vi "Finite_acq_gen_3.vi"(4 "Stimulator":T1={"frequency (Hz)"=1.0, "initial delay (ms)"=0.0, "# Stimuli"=0, "ON-OFF"=FALSE, "duty ratio"=0.0} {"frequency (Hz)" min=0.5 max=16.0 step=0.5 scale=0.0..10.0}, 5 "Shutter #2":T3={"Duration (ms)"=10.0, "Delay (ms)"=100.0, "# Cycles"=1, "period (ms)"=500.0, "ENABLE"=FALSE}, 6 "TRG detector":T2={"Delay (ms)"=100.0, "Duration (ms)"=1000.0, "ENABLE"=FALSE}, 7 "Shutter #1":T3={"Duration (ms)"=10.0, "Delay (ms)"=100.0, "# Cycles"=1, "period (ms)"=500.0, "ENABLE"=FALSE}, 8 "error in":errorcluster, 9 "samples per channel":i32=1000, 10 "ms/point":dbl=1.0, 11 "data":dbl[](array[numeric]) format="%0.2f") -> (3 "data 2":waveform(dbl)[](array[waveform]))   [LabVIEW 2011]
uses:
  <vilib>/DAQmx/write.llb/DAQmx Write (Analog 1D DBL 1Chan NSamp).vi
  <vilib>/DAQmx/read.llb/DAQmx Read (Analog 1D Wfm NChan NSamp).vi
  <vilib>/DAQmx/create/channels.llb/DAQmx Create Channel (AI-Voltage-Basic).vi
  <vilib>/DAQmx/configure/timing.llb/DAQmx Timing (Sample Clock).vi
  <vilib>/DAQmx/configure/trigger.llb/DAQmx Start Trigger (None).vi
  <vilib>/DAQmx/create/channels.llb/DAQmx Create Channel (CO-Pulse Generation-Frequency).vi
  <vilib>/DAQmx/configure/timing.llb/DAQmx Timing (Implicit).vi
  <vilib>/DAQmx/configure/trigger.llb/DAQmx Start Trigger (Digital Edge).vi
  <vilib>/DAQmx/create/channels.llb/DAQmx Create Channel (AO-Voltage-Basic).vi
  <vilib>/DAQmx/miscellaneous.llb/DAQmx Fill In Error Info.vi
  <vilib>/DAQmx/create/channels.llb/DAQmx Create Channel (CO-Pulse Generation-Time).vi
panel:
  # "STIMULATOR"
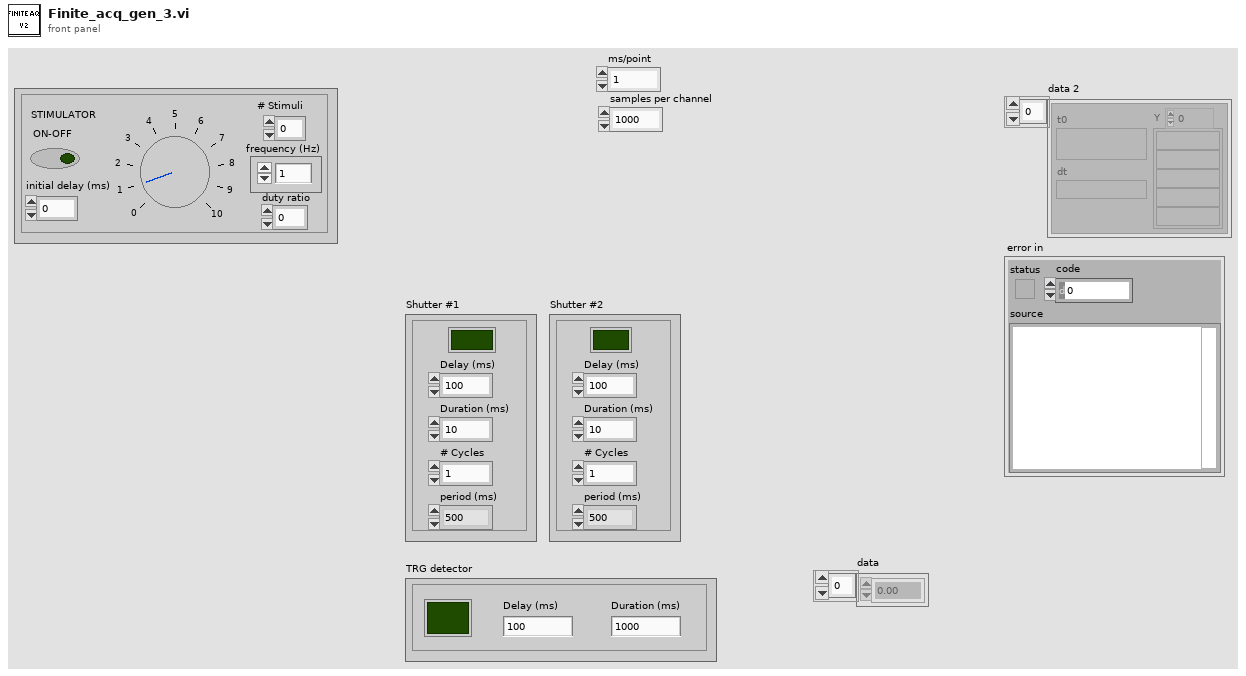
[diagram p1: front panel]
types:
  T1 = cluster{"frequency (Hz)":dbl, "initial delay (ms)":dbl, "# Stimuli":i8, "ON-OFF":bool, "duty ratio":dbl}
  T2 = cluster{"Delay (ms)":dbl, "Duration (ms)":dbl, "ENABLE":bool}
  T3 = cluster{"Duration (ms)":dbl, "Delay (ms)":dbl, "# Cycles":i8, "period (ms)":dbl, "ENABLE":bool}
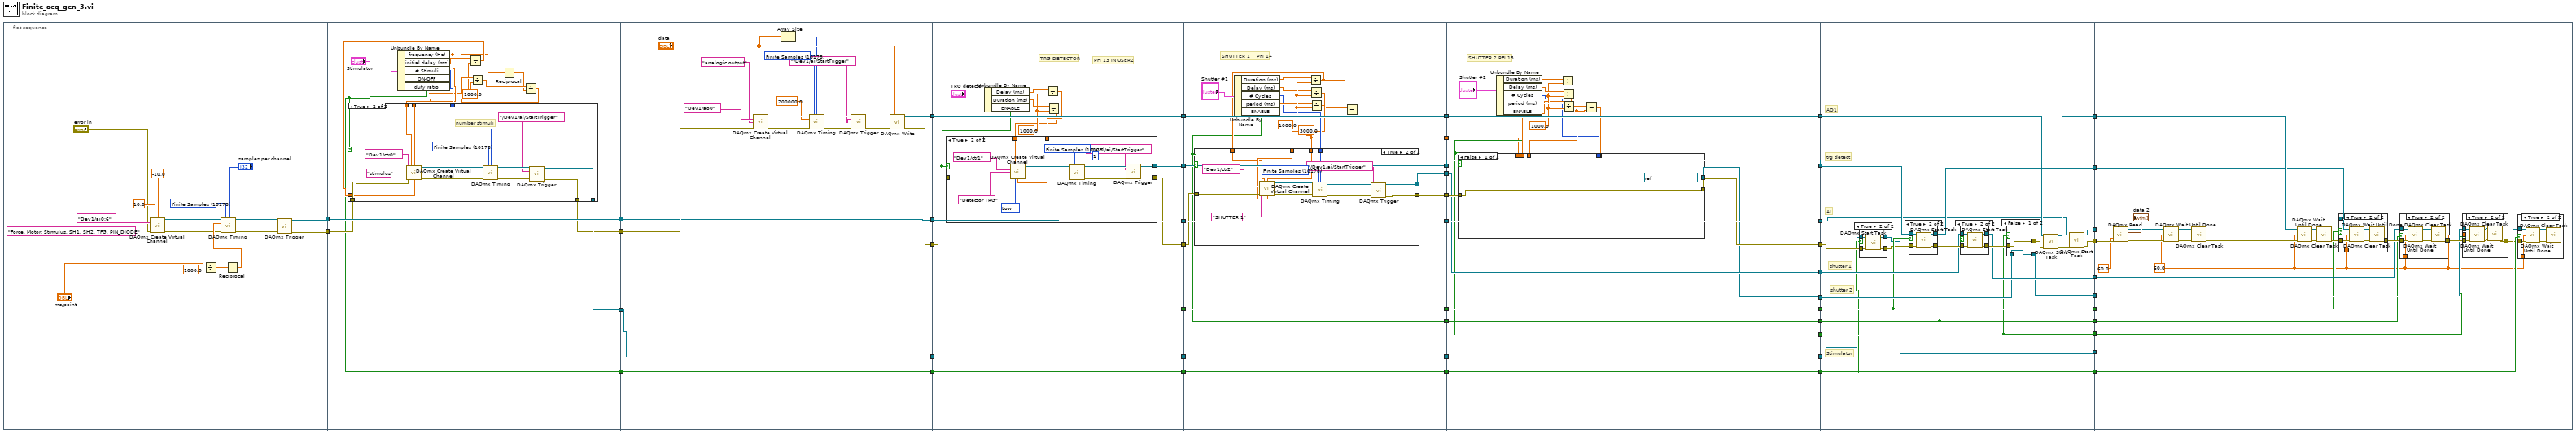
[diagram p0: block diagram]
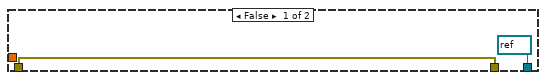
[diagram p2: hidden frame]
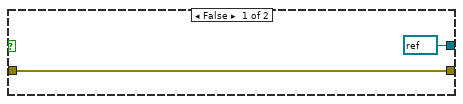
[diagram p3: hidden frame]
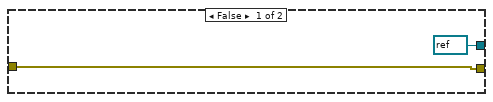
[diagram p4: hidden frame]
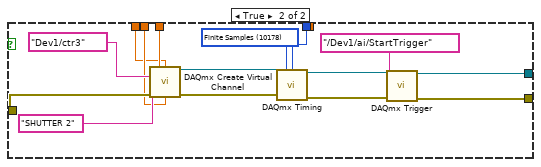
[diagram p5: hidden frame]
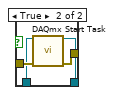
[diagram p7: hidden frame]
diagram:
  n1 = flat-sequence {
    tunnel: [w54] -> w16
    tunnel: [w52] -> w14
    tunnel: w16 -> [w81]
    tunnel: [w79] -> w15
    tunnel: w14 -> [w82]
    tunnel: [w82] -> w13
    tunnel: [w80] -> w8
    tunnel: [w75] -> w6
    tunnel: [w108] -> w48
    tunnel: [w113] -> w47
    tunnel: w15 -> [w109]
    tunnel: w13 -> [w108]
    tunnel: [w107] -> w46
    tunnel: [w101] -> w9
    tunnel: w8 -> [w101]
    tunnel: w6 -> [w100]
    tunnel: [w100] -> w5
    tunnel: w48 -> [w132]
    tunnel: [w132] -> w44
    tunnel: w47 -> [w128]
    tunnel: [w128] -> w43
    tunnel: w46 -> [w131]
    tunnel: [w130] -> w42
    tunnel: [w129] -> w41
    tunnel: [w121] -> w24
    tunnel: [w120] -> w10
    tunnel: w9 -> [w120]
    tunnel: w5 -> [w119]
    tunnel: [w119] -> w4
    tunnel: w44 -> [w169]
    tunnel: [w169] -> w40
    tunnel: w43 -> [w168]
    tunnel: [w168] -> w38
    tunnel: w42 -> [w166]
    tunnel: w41 -> [w167]
    tunnel: [w167] -> w35
    tunnel: [w165] -> w33
    tunnel: [w164] -> w31
    tunnel: [w154] -> w25
    tunnel: w24 -> [w154]
    tunnel: [w153] -> w23
    tunnel: [w152] -> w17
    tunnel: [w151] -> w11
    tunnel: w10 -> [w151]
    tunnel: w4 -> [w150]
    tunnel: [w150] -> w3
    tunnel: w40 -> [w209]
    tunnel: [w209] -> w39
    tunnel: w38 -> [w208]
    tunnel: [w208] -> w37
    tunnel: [w205] -> w36
    tunnel: w35 -> [w207]
    tunnel: [w207] -> w34
    tunnel: w33 -> [w206]
    tunnel: w31 -> [w204]
    tunnel: [w204] -> w30
    tunnel: [w203] -> w29
    tunnel: [w192] -> w26
    tunnel: w25 -> [w192]
    tunnel: w23 -> [w191]
    tunnel: [w191] -> w22
    tunnel: [w190] -> w21
    tunnel: w17 -> [w189]
    tunnel: [w188] -> w12
    tunnel: w11 -> [w188]
    tunnel: w3 -> [w187]
    tunnel: [w187] -> w2
    tunnel: w39 -> [w233]
    tunnel: w37 -> [w238]
    tunnel: [w237] -> w50
    tunnel: [w232] -> w49
    tunnel: w36 -> [w231]
    tunnel: w34 -> [w249]
    tunnel: [w248] -> w45
    tunnel: [w234] -> w32
    tunnel: w30 -> [w245]
    tunnel: w29 -> [w243]
    tunnel: [w244] -> w28
    tunnel: [w242] -> w27
    tunnel: w26 -> [w241]
    tunnel: w22 -> [w240]
    tunnel: w21 -> [w239]
    tunnel: [w241] -> w20
    tunnel: [w240] -> w19
    tunnel: [w239] -> w18
    tunnel: w12 -> [w229]
    tunnel: [w228] -> w7
    tunnel: w2 -> [w227]
    tunnel: [w227] -> w1
    tunnel: w50 -> [w290]
    tunnel: w49 -> [w296]
    tunnel: w45 -> [w284]
    tunnel: w32 -> [w297]
    tunnel: w28 -> [w283]
    tunnel: w27 -> [w282]
    tunnel: w20 -> [w281]
    tunnel: w19 -> [w280]
    tunnel: w18 -> [w279]
    tunnel: w7 -> [w277]
    tunnel: w1 -> [w276]
    frame #0 {
      w62 = 10178 items=["Finite Samples"=10178, "Continuous Samples"=10123, "Hardware Timed Single Point"=12522] ("sample mode")
      n2 = call-poly <vilib>:"DAQmx Create Virtual Channel.vi"("maximum value"=10.0, "minimum value"=-10.0, "physical channels"=tag "Dev1/ai0:6", "name to assign"="Force, Motor, Stimulus, SH1, SH2, TFG, PIN_DIODE", "error in"="error in") -> ("task out"=w61:refnum<k21>, "error out"=w60:errorcluster)  [unwired: 9 in]
      n3 = Divide(x="ms/point", y=1000.0) -> (x/y=w65:dbl)
      n4 = Reciprocal(x=w65) -> (1/x=w67:dbl)
      n5 = call-poly <vilib>:"DAQmx Timing.vi"("task/channels in"=w61, "sample mode"=w62, "samples per channel"="samples per channel", "rate"=w67, "error in"=w60) -> ("task out"=w53:refnum<k21>, "error out"=w55:errorcluster)  [unwired: 9 in]
      n6 = call-poly <vilib>:"DAQmx Trigger.vi"("task/channels in"=w53, "error in"=w55) -> ("task out"=w52:refnum<k21>, "error out"=w54:errorcluster)  [unwired: 12 in]
    }
    frame #1 {
      w71 = 1000.0 ("y")
      n7 = Unbundle By Name("Stimulator") -> ("frequency (Hz)"=w73:dbl, "initial delay (ms)"=w78:dbl, "# Stimuli"=w76:i8, "ON-OFF"=w75:bool, "duty ratio"=w72:dbl)
      n8 = Divide(x=w78, y=w71) -> (x/y=w77:dbl)
      n9 = Divide(x=w72, y=w71) -> (x/y=w70:dbl)
      n10 = Reciprocal(x=w73) -> (1/x=w69:dbl)
      n11 = Divide(x=w70, y=w69) -> (x/y=w68:dbl)
      n12 = case shown="True" w75 {
        tunnel: w81 -> [w84 w94]
        tunnel: [refnum<k21> refnum ("task out") w92] -> w80
        tunnel: [w84 w90] -> w79
        tunnel: w76 -> [_ w88]
        tunnel: w77 -> [_ w87]
        tunnel: w73 -> [_ w86]
        tunnel: w68 -> [_ w85]
        frame False {
        }
        frame True {
          w99 = 10178 items=["Finite Samples"=10178, "Continuous Samples"=10123, "Hardware Timed Single Point"=12522] ("sample mode")
          # "number stimuli"
          n13 = call-poly <vilib>:"DAQmx Create Virtual Channel.vi"("frequency"=w86, "duty cycle"=w85, "counter"=tag "Dev1/ctr0", "name to assign"="stimulus", "error in"=w94, "initial delay"=w87) -> ("task out"=w97:refnum<k21>, "error out"=w98:errorcluster)  [unwired: 8 in]
          n14 = call-poly <vilib>:"DAQmx Timing.vi"("task/channels in"=w97, "sample mode"=w99, "samples per channel"=w88, "error in"=w98) -> ("task out"=w93:refnum<k21>, "error out"=w91:errorcluster)  [unwired: 10 in]
          n15 = call-poly <vilib>:"DAQmx Trigger.vi"("task/channels in"=w93, "source"=tag "/Dev1/ai/StartTrigger", "error in"=w91) -> ("task out"=w92:refnum<k21>, "error out"=w90:errorcluster)  [unwired: 11 in]
        }
      }
    }
    frame #2 {
      w114 = 10178 items=["Finite Samples"=10178, "Continuous Samples"=10123, "Hardware Timed Single Point"=12522] ("sample mode")
      n16 = call-poly <vilib>:"DAQmx Create Virtual Channel.vi"("physical channels"=tag "Dev1/ao0", "name to assign"="analogic output", "error in"=w109) -> ("task out"=w117:refnum<k21>, "error out"=w116:errorcluster)  [unwired: 11 in]
      n17 = Array Size(array="data") -> (size(s)=w111:i32)
      n18 = call-poly <vilib>:"DAQmx Timing.vi"("task/channels in"=w117, "sample mode"=w114, "samples per channel"=w111, "rate"=200000.0, "error in"=w116) -> ("task out"=w106:refnum<k21>, "error out"=w104:errorcluster)  [unwired: 9 in]
      n19 = call-poly <vilib>:"DAQmx Trigger.vi"("task/channels in"=w106, "source"=tag "/Dev1/ai/StartTrigger", "error in"=w104) -> ("task out"=w105:refnum<k21>, "error out"=w103:errorcluster)  [unwired: 11 in]
      n20 = call-poly <vilib>:"DAQmx Write.vi"("task/channels in"=w105, "data"="data", "error in"=w103) -> ("task out"=w113:refnum<k21>, "error out"=w107:errorcluster)  [unwired: 10 in, 1 out]
    }
    frame #3 {
      w124 = 1000.0 ("y")
      # "PFI 13 IN USER2"
      # "TRG DETECTOR"
      n21 = Unbundle By Name("TRG detector") -> ("Delay (ms)"=w126:dbl, "Duration (ms)"=w125:dbl, "ENABLE"=w121:bool)
      n22 = Divide(x=w126, y=w124) -> (x/y=w123:dbl)
      n23 = Divide(x=w125, y=w124) -> (x/y=w122:dbl)
      n24 = case shown="True" w121 {
        tunnel: w131 -> [w134 w142]
        tunnel: [w134 w141] -> w130
        tunnel: [refnum<k21> refnum ("task out") w139] -> w129
        tunnel: w123 -> [_ w137]
        tunnel: w122 -> [_ w136]
        frame False {
        }
        frame True {
          w135 = 10214 items=["High"=10192, "Low"=10214] ("idle state")
          w145 = 10178 items=["Finite Samples"=10178, "Continuous Samples"=10123, "Hardware Timed Single Point"=12522] ("sample mode")
          n25 = call-poly <vilib>:"DAQmx Create Virtual Channel.vi"("high time"=w136, "counter"=tag "Dev1/ctr1", "name to assign"="Detector TRG", "error in"=w142, "idle state"=w135, "initial delay"=w137) -> ("task out"=w146:refnum<k21>, "error out"=w147:errorcluster)  [unwired: 8 in]
          n26 = call-poly <vilib>:"DAQmx Timing.vi"("task/channels in"=w146, "sample mode"=w145, "samples per channel"=1, "error in"=w147) -> ("task out"=w149:refnum<k21>, "error out"=w148:errorcluster)  [unwired: 10 in]
          n27 = call-poly <vilib>:"DAQmx Trigger.vi"("task/channels in"=w149, "source"=tag "/Dev1/ai/StartTrigger", "error in"=w148) -> ("task out"=w139:refnum<k21>, "error out"=w141:errorcluster)  [unwired: 11 in]
        }
      }
    }
    frame #4 {
      w152 = 3000.0
      w162 = 1000.0 ("y")
      # "SHUTTER 1    PFI 14"
      n28 = Unbundle By Name("Shutter #1") -> ("Duration (ms)"=w161:dbl, "Delay (ms)"=w160:dbl, "# Cycles"=w158:i8, "period (ms)"=w159:dbl, "ENABLE"=w153:bool)
      n29 = Divide(x=w161, y=w162) -> (x/y=w155:dbl)
      n30 = Divide(x=w160, y=w162) -> (x/y=w157:dbl)
      n31 = case shown="True" w153 {
        tunnel: w166 -> [w171 w184]
        tunnel: [w171 w177] -> w165
        tunnel: [refnum<k21> refnum ("task out") w176] -> w164
        tunnel: w158 -> [_ w175]
        tunnel: w157 -> [_ w174]
        tunnel: w155 -> [_ w173]
        tunnel: w152 -> [_ w172]
        frame False {
        }
        frame True {
          w178 = 10178 items=["Finite Samples"=10178, "Continuous Samples"=10123, "Hardware Timed Single Point"=12522] ("sample mode")
          n32 = call-poly <vilib>:"DAQmx Create Virtual Channel.vi"("high time"=w173, "low time"=w172, "counter"=tag "Dev1/ctr2", "name to assign"="SHUTTER 1", "error in"=w184, "initial delay"=w174) -> ("task out"=w180:refnum<k21>, "error out"=w183:errorcluster)  [unwired: 8 in]
          n33 = call-poly <vilib>:"DAQmx Timing.vi"("task/channels in"=w180, "sample mode"=w178, "samples per channel"=w175, "error in"=w183) -> ("task out"=w179:refnum<k21>, "error out"=w182:errorcluster)  [unwired: 10 in]
          n34 = call-poly <vilib>:"DAQmx Trigger.vi"("task/channels in"=w179, "source"=tag "/Dev1/ai/StartTrigger", "error in"=w182) -> ("task out"=w176:refnum<k21>, "error out"=w177:errorcluster)  [unwired: 11 in]
        }
      }
      n35 = Divide(x=w159, y=w162) -> (x/y=w156:dbl)
      n36 = Subtract(x=w156, y=w155) -> ()  [unwired: 1 out]
    }
    frame #5 {
      w198 = 1000.0 ("y")
      # "SHUTTER 2 PFI 15"
      n37 = Unbundle By Name("Shutter #2") -> ("Duration (ms)"=w201:dbl, "Delay (ms)"=w200:dbl, "# Cycles"=w193:i8, "period (ms)"=w199:dbl, "ENABLE"=w190:bool)
      n38 = Divide(x=w201, y=w198) -> (x/y=w196:dbl)
      n39 = Divide(x=w200, y=w198) -> (x/y=w194:dbl)
      n40 = Divide(x=w199, y=w198) -> (x/y=w197:dbl)
      n41 = Subtract(x=w197, y=w196) -> (x-y=w195:dbl)
      n42 = case shown="False" w190 {
        tunnel: w206 -> [w211 w223]
        tunnel: [w211 w222] -> w205
        tunnel: [refnum<k21> refnum ("task out") w221] -> w203
        tunnel: w196 -> [_ w215]
        tunnel: w195 -> [_ _]
        tunnel: w194 -> [_ w214]
        tunnel: w193 -> [_ w213]
        tunnel: w189 -> [_ w212]
        frame False {
        }
        frame True {
          w216 = 10178 items=["Finite Samples"=10178, "Continuous Samples"=10123, "Hardware Timed Single Point"=12522] ("sample mode")
          n43 = call-poly <vilib>:"DAQmx Create Virtual Channel.vi"("high time"=w215, "low time"=w212, "counter"=tag "Dev1/ctr3", "name to assign"="SHUTTER 2", "error in"=w223, "initial delay"=w214) -> ("task out"=w220:refnum<k21>, "error out"=w218:errorcluster)  [unwired: 8 in]
          n44 = call-poly <vilib>:"DAQmx Timing.vi"("task/channels in"=w220, "sample mode"=w216, "samples per channel"=w213, "error in"=w218) -> ("task out"=w219:refnum<k21>, "error out"=w217:errorcluster)  [unwired: 10 in]
          n45 = call-poly <vilib>:"DAQmx Trigger.vi"("task/channels in"=w219, "source"=tag "/Dev1/ai/StartTrigger", "error in"=w217) -> ("task out"=w221:refnum<k21>, "error out"=w222:errorcluster)  [unwired: 11 in]
        }
      }
    }
    frame #6 {
      # "Stimulator"
      # "shutter 2"
      # "shutter 1"
      # "trg detect"
      # "AO1"
      # "AI"
      n46 = case shown="True" w227 {
        tunnel: w231 -> [w250 w255]
        tunnel: w229 -> [w251 w254]
        tunnel: [w251 w253] -> w228
        tunnel: [w250 w252] -> w230
        frame False {
        }
        frame True {
          n47 = call <vilib>:"DAQmx Start Task.vi"("task/channels in"=w254, "error in"=w255) -> ("task out"=w253:refnum<k21>, "error out"=w252:errorcluster)  [unwired: 12 in]
        }
      }
      n48 = case shown="True" w241 {
        tunnel: w230 -> [w268 w273]
        tunnel: w249 -> [w269 w272]
        tunnel: [w269 w271] -> w248
        tunnel: [w268 w270] -> w247
        frame False {
        }
        frame True {
          n49 = call <vilib>:"DAQmx Start Task.vi"("task/channels in"=w272, "error in"=w273) -> ("task out"=w271:refnum<k21>, "error out"=w270:errorcluster)  [unwired: 12 in]
        }
      }
      n50 = case shown="True" w240 {
        tunnel: w247 -> [w263 w267]
        tunnel: [w263 w266] -> w246
        tunnel: w245 -> [w262 w265]
        tunnel: [w262 w264] -> w244
        frame False {
        }
        frame True {
          n51 = call <vilib>:"DAQmx Start Task.vi"("task/channels in"=w265, "error in"=w267) -> ("task out"=w264:refnum<k21>, "error out"=w266:errorcluster)  [unwired: 12 in]
        }
      }
      n52 = case shown="False" w239 {
        tunnel: w246 -> [w257 w261]
        tunnel: [w257 w260] -> w236
        tunnel: w243 -> [w256 w259]
        tunnel: [w256 w258] -> w242
        frame False {
        }
        frame True {
          n53 = call <vilib>:"DAQmx Start Task.vi"("task/channels in"=w259, "error in"=w261) -> ("task out"=w258:refnum<k21>, "error out"=w260:errorcluster)  [unwired: 12 in]
        }
      }
      n54 = call <vilib>:"DAQmx Start Task.vi"("task/channels in"=w238, "error in"=w236) -> ("task out"=w237:refnum<k21>, "error out"=w235:errorcluster)  [unwired: 12 in]
      n55 = call <vilib>:"DAQmx Start Task.vi"("task/channels in"=w233, "error in"=w235) -> ("task out"=w232:refnum<k21>, "error out"=w234:errorcluster)  [unwired: 12 in]
    }
    frame #7 {
      w274 = 60.0 ("timeout (sec)")
      n56 = call-poly <vilib>:"DAQmx Read.vi"("task/channels in"=w296, "timeout"=60.0, "error in"=w297) -> ("task out"=w295:refnum<k21>, "data"=→"data 2":waveform(dbl)[], "error out"=w292:errorcluster)  [unwired: 10 in]
      n57 = call <vilib>:"DAQmx Wait Until Done.vi"("task/channels in"=w295, "timeout (sec)"=w274, "error in"=w292) -> ("task out"=w293:refnum<k21>, "error out"=w294:errorcluster)  [unwired: 11 in]
      n58 = call <vilib>:"DAQmx Clear Task.vi"("task in"=w293, "error in"=w294) -> ("error out"=w291:errorcluster)  [unwired: 13 in]
      n59 = call <vilib>:"DAQmx Wait Until Done.vi"("task/channels in"=w290, "timeout (sec)"=w274, "error in"=w291) -> ("task out"=w289:refnum<k21>, "error out"=w288:errorcluster)  [unwired: 11 in]
      n60 = call <vilib>:"DAQmx Clear Task.vi"("task in"=w289, "error in"=w288) -> ("error out"=w287:errorcluster)  [unwired: 13 in]
      n61 = case shown="True" w281 {
        tunnel: w287 -> [w318 w324]
        tunnel: [w318 w322] -> w286
        tunnel: w284 -> [_ w321]
        tunnel: w274 -> [_ w319]
        frame False {
        }
        frame True {
          n62 = call <vilib>:"DAQmx Wait Until Done.vi"("task/channels in"=w321, "timeout (sec)"=w319, "error in"=w324) -> ("task out"=w320:refnum<k21>, "error out"=w323:errorcluster)  [unwired: 11 in]
          n63 = call <vilib>:"DAQmx Clear Task.vi"("task in"=w320, "error in"=w323) -> ("error out"=w322:errorcluster)  [unwired: 13 in]
        }
      }
      n64 = case shown="True" w280 {
        tunnel: w286 -> [w311 w317]
        tunnel: [w311 w315] -> w285
        tunnel: w283 -> [_ w314]
        tunnel: w274 -> [_ w312]
        frame False {
        }
        frame True {
          n65 = call <vilib>:"DAQmx Wait Until Done.vi"("task/channels in"=w314, "timeout (sec)"=w312, "error in"=w317) -> ("task out"=w313:refnum<k21>, "error out"=w316:errorcluster)  [unwired: 11 in]
          n66 = call <vilib>:"DAQmx Clear Task.vi"("task in"=w313, "error in"=w316) -> ("error out"=w315:errorcluster)  [unwired: 13 in]
        }
      }
      n67 = case shown="True" w279 {
        tunnel: w285 -> [w304 w310]
        tunnel: w282 -> [_ w308]
        tunnel: w274 -> [_ w306]
        tunnel: [w304 w305] -> w275
        frame False {
        }
        frame True {
          n68 = call <vilib>:"DAQmx Wait Until Done.vi"("task/channels in"=w308, "timeout (sec)"=w306, "error in"=w310) -> ("task out"=w307:refnum<k21>, "error out"=w309:errorcluster)  [unwired: 11 in]
          n69 = call <vilib>:"DAQmx Clear Task.vi"("task in"=w307, "error in"=w309) -> ("error out"=w305:errorcluster)  [unwired: 13 in]
        }
      }
      n70 = case shown="True" w276 {
        tunnel: w275 -> [_ w303]
        tunnel: w277 -> [_ w301]
        tunnel: w274 -> [_ w299]
        frame False {
        }
        frame True {
          n71 = call <vilib>:"DAQmx Wait Until Done.vi"("task/channels in"=w301, "timeout (sec)"=w299, "error in"=w303) -> ("task out"=w300:refnum<k21>, "error out"=w302:errorcluster)  [unwired: 11 in]
          n72 = call <vilib>:"DAQmx Clear Task.vi"("task in"=w300, "error in"=w302) -> ()  [unwired: 13 in, 1 out]
        }
      }
    }
  }
